vi "SubVICreator.vi"(2 "X1":dbl, 3 "X2":dbl, 4 "Y1":dbl) -> (1 "M":dbl)   [LabVIEW 2023]
panel:
  in  "Y2":dbl
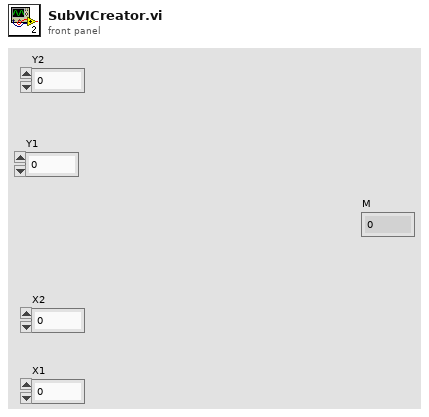
[diagram p1: front panel]
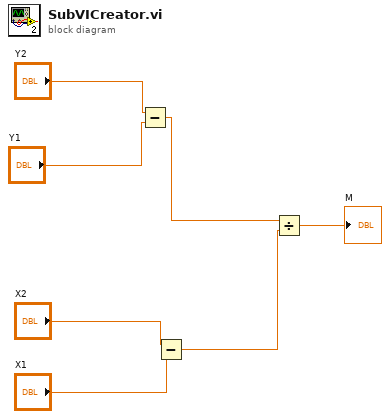
[diagram p0: block diagram]
diagram:
  n1 = Subtract(x="Y2", y="Y1") -> (x-y=w2:dbl)
  n2 = Subtract(x="X2", y="X1") -> (x-y=w3:dbl)
  n3 = Divide(x=w2, y=w3) -> (x/y=→"M":dbl)
